vi "Test Properties Report (XML).vi"() -> ()   [LabVIEW 2013]
uses:
  classes/Test Result/Node Results (Extended).ctl
  classes/Test Result/Test Node (Extended).ctl
  classes/Test Result/Test Registration Data.ctl
  classes/Test Result/Assert Event Data (Extended).ctl
  classes/Test Suite/Test Suite.lvclass
  classes/Test Result/Test Result.lvclass
panel:
  out "Test Results":T1[](array[typedef])
  in  "error in (no error)":errorcluster
  out "error out":errorcluster
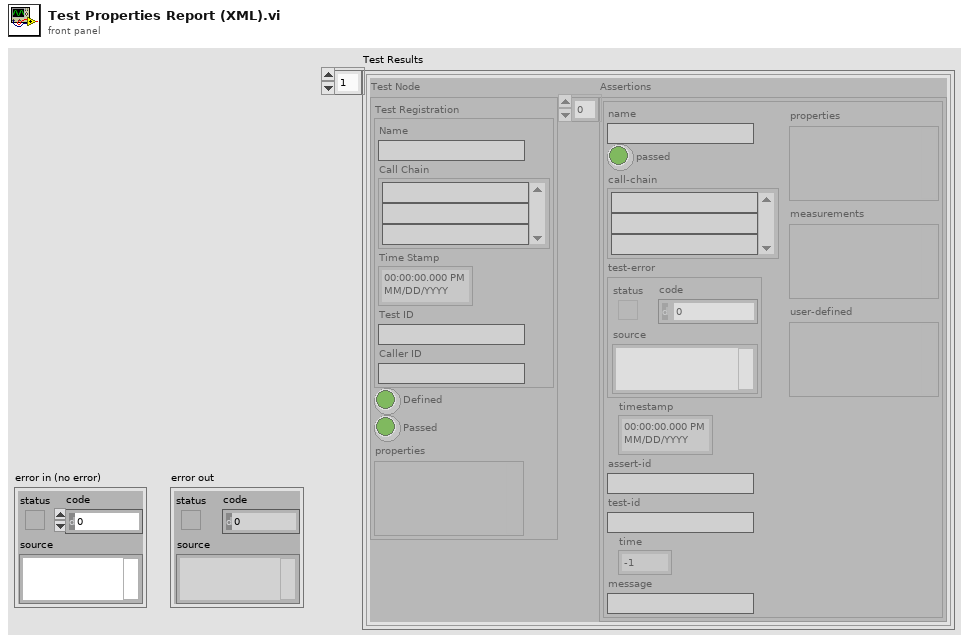
[diagram p1: front panel]
types:
  T1 = typedef "Caraya.lvlib/Test Result.lvclass/Node Results (Extended).ctl" = cluster{"Test Node":T2, "Assertions":T4[]}
  T2 = typedef "Caraya.lvlib/Test Result.lvclass/Test Node (Extended).ctl" = cluster{"Test Registration":T3, "Defined":bool, "Passed":bool, "properties":variant}
  T3 = typedef "Caraya.lvlib/Test Result.lvclass/Test Registration Data.ctl" = cluster{"Name":string, "Call Chain":string[], "Time Stamp":timestamp, "Test ID":string, "Caller ID":string}
  T4 = typedef "Caraya.lvlib/Test Result.lvclass/Assert Event Data (Extended).ctl" = cluster{"name":string, "passed":bool, "call-chain":string[], "test-error":errorcluster, "timestamp":timestamp, "assert-id":string, "test-id":string, "time":dbl, "message":string, "properties":variant, "measurements":variant, "user-defined":variant}
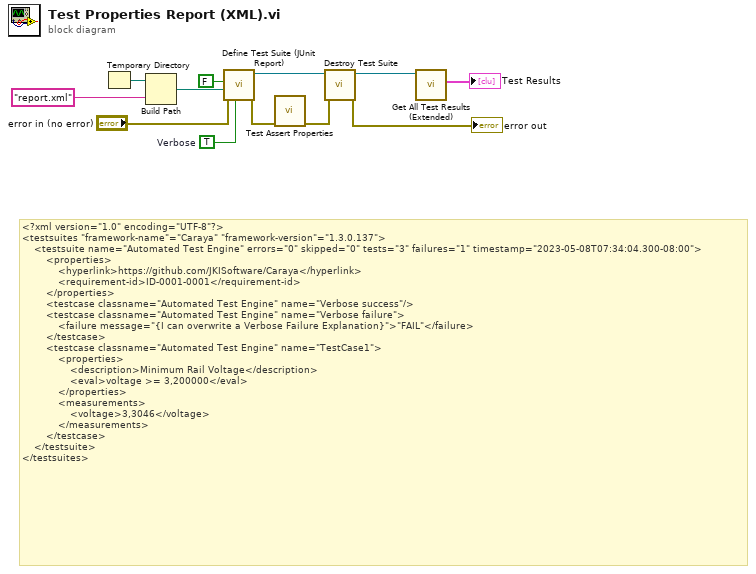
[diagram p0: block diagram]
diagram:
  w3 = TRUE  # Verbose
  # "<?xml version=\"1.0\" encoding=\"UTF-8\"?>\n<testsuites \"framework-name\"=\"Caraya\" \"framework-version\"=\"1.3.0.137\">\n    <testsuite name=\"Automated Test Engine\" errors=\"0\" skipped=\"0\" tests=\"3\" failures=\"1\" timestamp=\"2023-05-08T07:34:04.300-08:00\">\n        <properties>\n            <hyperlink>https://github.com/JKISoftware/Caraya</hyperlink>\n            <requirement-id>ID-0001-0001</requirement-id>\n        </properties>\n        <testcase classname=\"Automated Test Engine\" name=\"Verbose success\"/>\n        <testcase classname=\"Automated Test Engine\" name=\"Verbose failure\">\n            <failure message=\"{I can overwrite a Verbose Failure Explanation}\">\"FAIL\"</failure>\n        </testcase>\n        <testcase classname=\"Automated Test Engine\" name=\"TestCase1\">\n            <properties>\n                <description>Minimum Rail Voltage</description>\n                <eval>voltage >= 3,200000</eval>\n            </properties>\n            <measurements>\n                <voltage>3,3046</voltage>\n            </measurements>\n        </testcase>\n    </testsuite>\n</testsuites>"
  n1 = Temporary Directory() -> (w12:path)
  n2 = Build Path(base path=w12, name or relative path="report.xml") -> (appended path=w2:path)
  n3 = call "Define Test Suite (JUnit Report).vi"("Verbose (F)"=w3, "error in (no error)"="error in (no error)", "Report Path"=w2, "Interactive"=FALSE) -> ("error out"=w5:errorcluster, "Test Suite"=w4:refnum<class "Test Suite.lvclass">)  [unwired: 5 in, 1 out]
  n4 = call "Test Assert Properties.vi"("error in (no error)"=w5) -> ("error out"=w9:errorcluster)  [unwired: 10 in]
  n5 = call-dynamic "Destroy Test Suite.vi"("error in (no error)"=w9, "Test Suite in"=w4) -> ("error out"=→"error out":errorcluster, "Test Suite Results"=w11:refnum<class "Test Result.lvclass">)  [unwired: 8 in]
  n6 = call "Get All Test Results (Extended).vi"("Test Result in"=w11) -> ("Test Results"=→"Test Results":T1[])  [unwired: 8 in, 2 out]
